vi "开关机和泵.vi"() -> ()   [LabVIEW 2013]
panel:
  in  "Stopprogram":bool
  in  "Gate":bool
  out "PumpSpeed":u8
  out "PumpTemp":u16
  out "PumpKW":dbl
  out "PumpAmps":dbl
  out "PumpVolts":dbl
  out "LenseHVSet":dbl
  out "PulseHVSet":dbl
  out "TarHVSet":dbl
  out "MCPHVSet":dbl
  in  "LenseHV":dbl
  in  "PulseHV":dbl
  in  "TarHV":dbl
  in  "MCPHV":dbl
  in  "SopPump":bool
  in  "StartPump":bool
  in  "ConfiguredPumpCom":refnum<visa-resource-name>
  in  "Main_Samp":bool
  in  "Samp_Atmos":bool
  in  "Turbo_Fore":bool
  in  "LowPressure":dbl
  in  "Startsystem":bool
  # "GetAI"
  # "SetAO"
  # "GetDI"
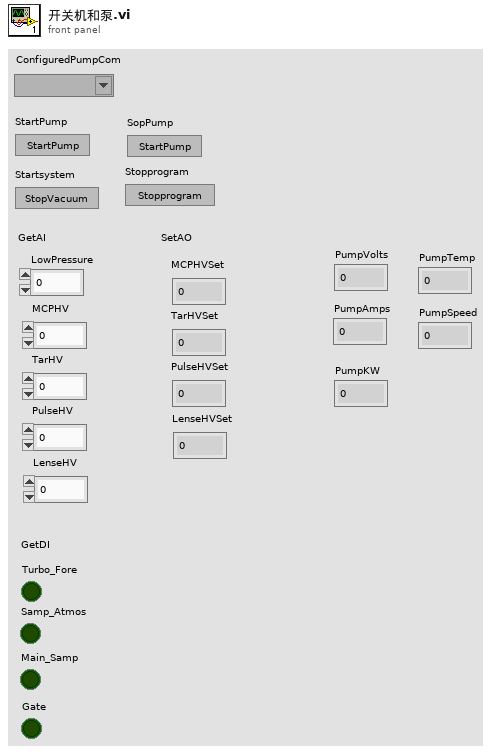
[diagram p1: front panel]
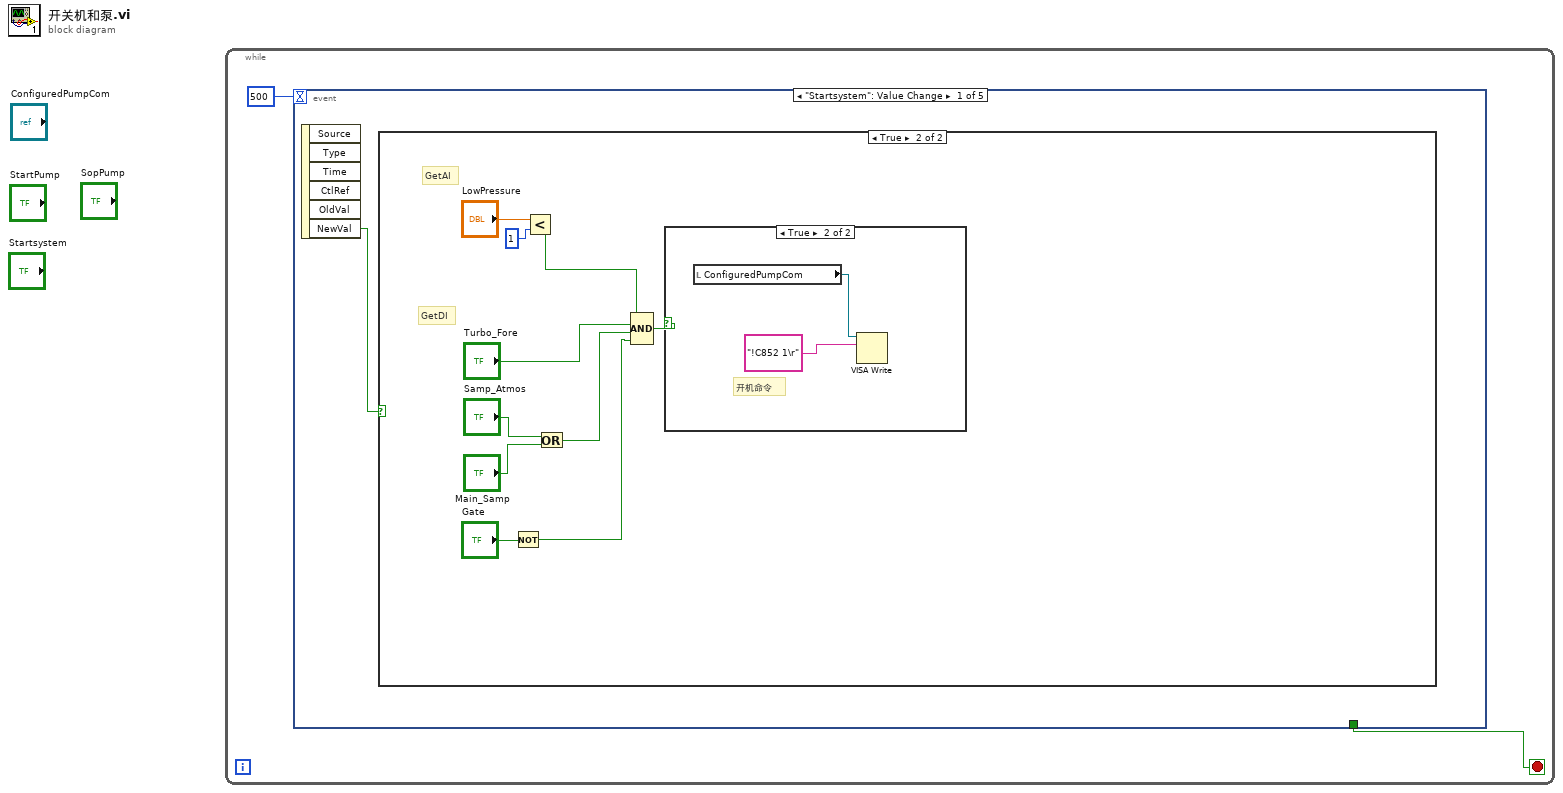
[diagram p0: block diagram]
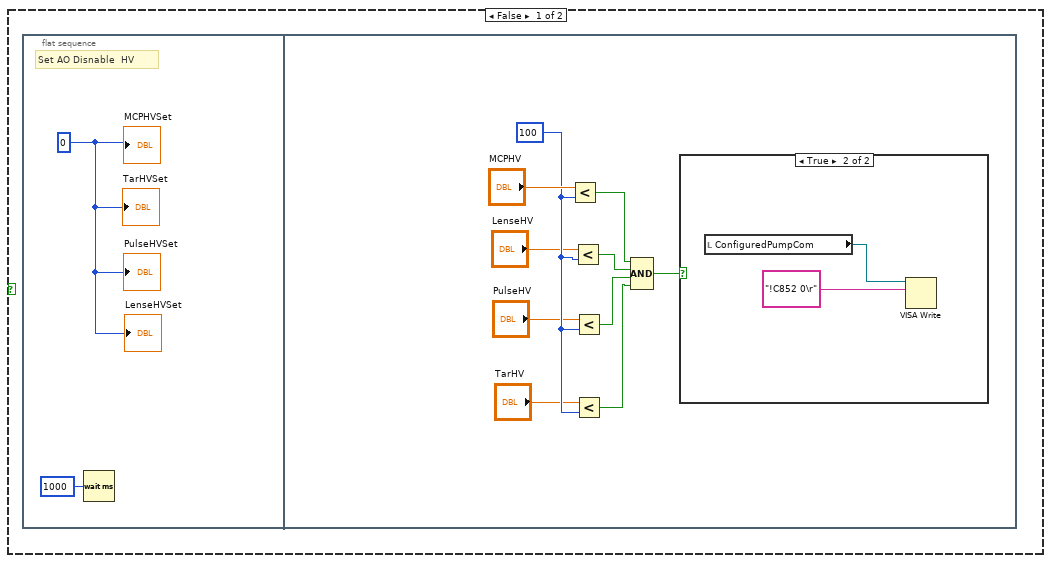
[diagram p2: hidden frame]
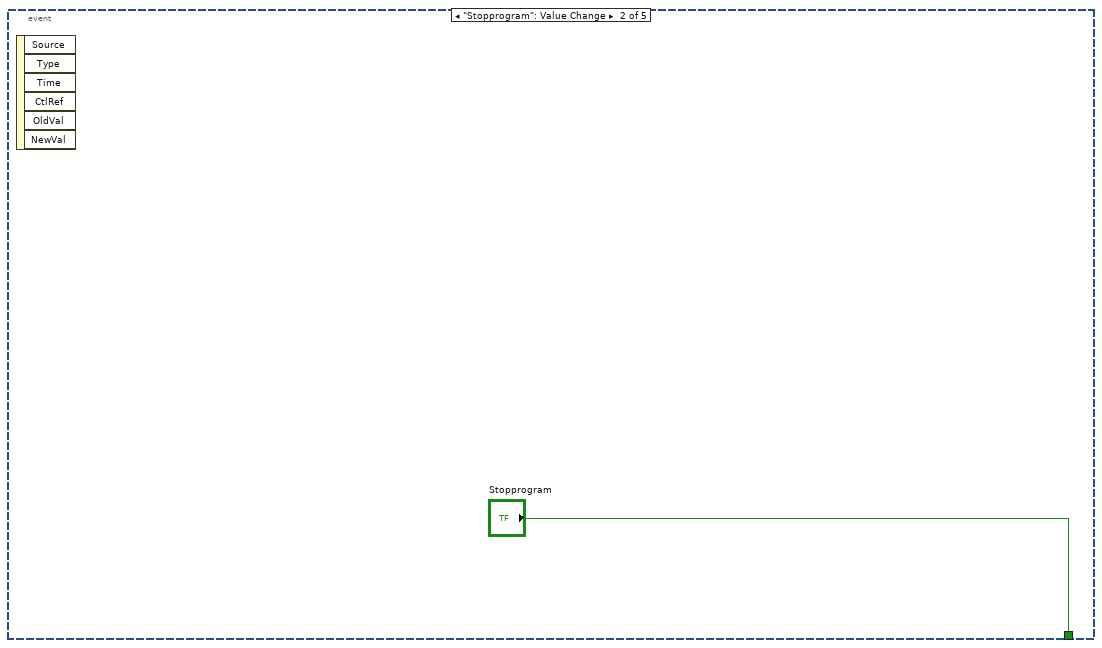
[diagram p5: hidden frame]
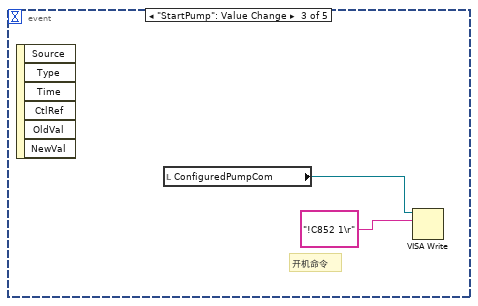
[diagram p6: hidden frame]
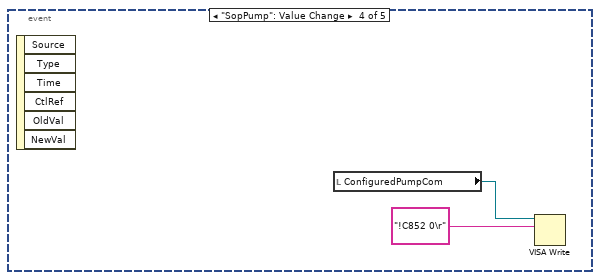
[diagram p7: hidden frame]
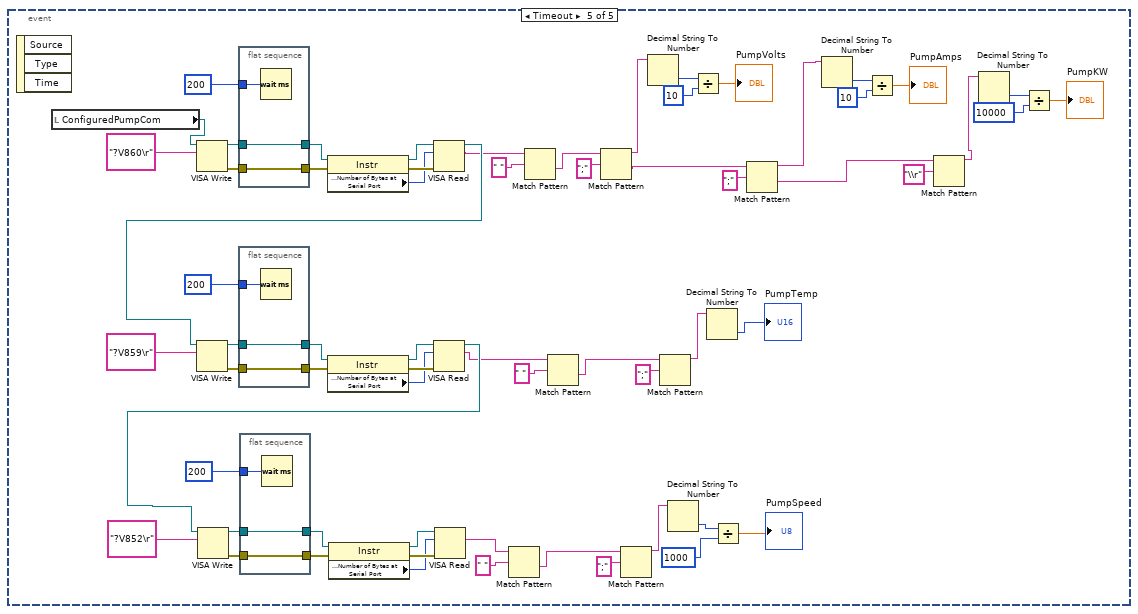
[diagram p8: hidden frame]
diagram:
  n1 = while {
    stop <- w1 stop-if-true
    n2 = event shown="[0] \"Startsystem\": Value Change" {
      selector: _ -> [_ _ _ _ _]
      dyn-events: _ -> [_ _ _ _ _]
      timeout: 500 -> [_ _ _ _ _]
      tunnel: [_ "Stopprogram" _ _ _] -> w1
      event "Startsystem": Value Change {
        n3 = event-data() -> ("NewVal"=w3:bool)  [unwired: 1 in, 5 out]
        n4 = case shown="True" w3 {
          frame False {
            n5 = flat-sequence {
              frame #0 {
                w5 = 0
                # "Set AO Disnable  HV"
                n6 = Wait (ms)(milliseconds to wait=u32 1000) -> ()  [unwired: 1 out]
                "MCPHVSet" <- w5
                "TarHVSet" <- w5
                "PulseHVSet" <- w5
                "LenseHVSet" <- w5
              }
              frame #1 {
                w14 = 100
                n7 = Less?(x="MCPHV", y=w14) -> (x < y?=w10:bool)
                n8 = Less?(x="LenseHV", y=w14) -> (x < y?=w9:bool)
                n9 = Less?(x="PulseHV", y=w14) -> (x < y?=w8:bool)
                n10 = Less?(x="TarHV", y=w14) -> (x < y?=w7:bool)
                n11 = Compound Arithmetic op=AND(w10, w9, w8, w7) -> (w6:bool)
                n12 = case shown="True" w6 {
                  frame False {
                  }
                  frame True {
                    n13 = local read "ConfiguredPumpCom"() -> (w16:refnum<visa-resource-name>)
                    n14 = VISA Write(VISA resource name=w16, write buffer="!C852 0\r" ("Command")) -> ()  [unwired: 1 in, 3 out]
                  }
                }
              }
            }
          }
          frame True {
            # "GetAI"
            # "GetDI"
            n15 = Not(x="Gate") -> (.not. x?=w18:bool)
            n16 = Less?(x="LowPressure", y=1) -> (x < y?=w23:bool)
            n17 = Or(x="Samp_Atmos", y="Main_Samp") -> (x .or. y?=w21:bool)
            n18 = Compound Arithmetic op=AND(w23, "Turbo_Fore", w21, w18) -> (w20:bool)
            n19 = case shown="True" w20 {
              frame False {
              }
              frame True {
                # "开机命令"
                n20 = local read "ConfiguredPumpCom"() -> (w28:refnum<visa-resource-name>)
                n21 = VISA Write(VISA resource name=w28, write buffer="!C852 1\r" ("Command")) -> ()  [unwired: 1 in, 3 out]
              }
            }
          }
        }
      }
      event "Stopprogram": Value Change {
        n22 = event-data() -> ()  [unwired: 1 in, 6 out]
      }
      event "StartPump": Value Change {
        # "开机命令"
        n23 = event-data() -> ()  [unwired: 1 in, 6 out]
        n24 = local read "ConfiguredPumpCom"() -> (w31:refnum<visa-resource-name>)
        n25 = VISA Write(VISA resource name=w31, write buffer="!C852 1\r" ("Command")) -> ()  [unwired: 1 in, 3 out]
      }
      event "SopPump": Value Change {
        n26 = event-data() -> ()  [unwired: 1 in, 6 out]
        n27 = local read "ConfiguredPumpCom"() -> (w34:refnum<visa-resource-name>)
        n28 = VISA Write(VISA resource name=w34, write buffer="!C852 0\r" ("Command")) -> ()  [unwired: 1 in, 3 out]
      }
      event Timeout {
        n29 = event-data() -> ()  [unwired: 1 in, 3 out]
        n30 = local read "ConfiguredPumpCom"() -> (w47:refnum<visa-resource-name>)
        n31 = VISA Write(VISA resource name=w47, write buffer="?V860\r" ("Command")) -> (VISA resource name out=w41:refnum<visa-resource-name>, error out=w43:errorcluster)  [unwired: 1 in, 1 out]
        n32 = flat-sequence {
          tunnel: w43 -> [w106]
          tunnel: [w106] -> w42
          tunnel: w41 -> [w105]
          tunnel: [w105] -> w40
          tunnel: u32 200 ("delay before read (ms)") -> [w107]
          frame #0 {
            n33 = Wait (ms)(milliseconds to wait=w107) -> ()  [unwired: 1 out]
          }
        }
        n34 = flat-sequence {
          tunnel: w73 -> [w103]
          tunnel: [w103] -> w72
          tunnel: w71 -> [w102]
          tunnel: [w102] -> w70
          tunnel: u32 200 ("delay before read (ms)") -> [w104]
          frame #0 {
            n35 = Wait (ms)(milliseconds to wait=w104) -> ()  [unwired: 1 out]
          }
        }
        n36 = flat-sequence {
          tunnel: w89 -> [w100]
          tunnel: [w100] -> w88
          tunnel: w87 -> [w99]
          tunnel: [w99] -> w86
          tunnel: u32 200 ("delay before read (ms)") -> [w101]
          frame #0 {
            n37 = Wait (ms)(milliseconds to wait=w101) -> ()  [unwired: 1 out]
          }
        }
        n38 = property class="Instr"(reference=w40, error in=w42) -> (reference out=w38:refnum<visa-resource-name>, error out=w37:errorcluster, "Serial Settings:Number of Bytes at Serial Port"=w36:u32)
        n39 = property class="Instr"(reference=w70, error in=w72) -> (reference out=w68:refnum<visa-resource-name>, error out=w67:errorcluster, "Serial Settings:Number of Bytes at Serial Port"=w66:u32)
        n40 = property class="Instr"(reference=w86, error in=w88) -> (reference out=w84:refnum<visa-resource-name>, error out=w83:errorcluster, "Serial Settings:Number of Bytes at Serial Port"=w82:u32)
        n41 = VISA Read(VISA resource name=w38, byte count=w36, error in (no error)=w37) -> (VISA resource name out=w74:refnum<visa-resource-name>, read buffer=w54:string)  [unwired: 2 out]
        n42 = VISA Write(VISA resource name=w74, write buffer="?V859\r" ("Command")) -> (VISA resource name out=w71:refnum<visa-resource-name>, error out=w73:errorcluster)  [unwired: 1 in, 1 out]
        n43 = VISA Read(VISA resource name=w68, byte count=w66, error in (no error)=w67) -> (VISA resource name out=w90:refnum<visa-resource-name>, read buffer=w79:string)  [unwired: 2 out]
        n44 = VISA Write(VISA resource name=w90, write buffer="?V852\r" ("Command")) -> (VISA resource name out=w87:refnum<visa-resource-name>, error out=w89:errorcluster)  [unwired: 1 in, 1 out]
        n45 = VISA Read(VISA resource name=w84, byte count=w82, error in (no error)=w83) -> (read buffer=w95:string)  [unwired: 3 out]
        n46 = Match Pattern(string=w95, regular expression=" ") -> (after substring=w92:string)  [unwired: 1 in, 3 out]
        n47 = Match Pattern(string=w54, regular expression=" ") -> (after substring=w56:string)  [unwired: 1 in, 3 out]
        n48 = Match Pattern(string=w79, regular expression=" ") -> (after substring=w76:string)  [unwired: 1 in, 3 out]
        n49 = Match Pattern(string=w56, regular expression=";") -> (before substring=w58:string, after substring=w60:string)  [unwired: 1 in, 2 out]
        n50 = Match Pattern(string=w92, regular expression=";") -> (before substring=w94:string)  [unwired: 1 in, 3 out]
        n51 = Decimal String To Number(string=w58) -> (number=w44:i32)  [unwired: 2 in, 1 out]
        n52 = Match Pattern(string=w76, regular expression=";") -> (before substring=w78:string)  [unwired: 1 in, 3 out]
        n53 = Decimal String To Number(string=w94) -> (number=w96:i32)  [unwired: 2 in, 1 out]
        n54 = Divide(x=w44, y=10) -> (x/y=→"PumpVolts":dbl)
        n55 = Decimal String To Number(string=w78) -> (number=→"PumpTemp":i32)  [unwired: 2 in, 1 out]
        n56 = Divide(x=w96, y=1000) -> (x/y=→"PumpSpeed":dbl)
        n57 = Match Pattern(string=w60, regular expression=";") -> (before substring=w61:string, after substring=w63:string)  [unwired: 1 in, 2 out]
        n58 = Decimal String To Number(string=w61) -> (number=w48:i32)  [unwired: 2 in, 1 out]
        n59 = Divide(x=w48, y=10) -> (x/y=→"PumpAmps":dbl)
        n60 = Match Pattern(string=w63, regular expression="\\r") -> (before substring=w64:string)  [unwired: 1 in, 3 out]
        n61 = Decimal String To Number(string=w64) -> (number=w51:i32)  [unwired: 2 in, 1 out]
        n62 = Divide(x=w51, y=10000) -> (x/y=→"PumpKW":dbl)
      }
    }
  }
